vi "Exercise 2.1 DHTxx.vi"() -> ()   [LabVIEW 2014]
uses:
  <vilib>/Q-Wave Systems/QwaveSys RPi Training Package (Demo)/Addons/QwaveSys RPi Training Library.lvlib
  <vilib>/RAFA Solutions/Wooden UI Controls Kit Library Light/Graph/XY Graph.ctl
  <vilib>/RAFA Solutions/Wooden UI Controls Kit Library Light/Wooden UI Controls Kit Library Light.lvlib
  <vilib>/RAFA Solutions/Wooden UI Controls Kit Library Light/Numeric/Numeric Indicator.ctl
  <vilib>/RAFA Solutions/Rainbow Flat UI Controls Kit (Light)/Numeric/Thermometer.ctl
  <vilib>/RAFA Solutions/Rainbow Flat UI Controls Kit (Light)/Rainbow Light.lvlib
  <vilib>/RAFA Solutions/Rainbow Flat UI Controls Kit (Light)/Graph/XY Graph.ctl
panel:
  out "Waveform Chart":sgl(graph) caption="F  Chart 2"
  out "F Meter 2":dbl(knob) scale=0.0..100.0
  out "H & C Graph":T1
  out "C Chart":sgl(graph)
  out "H Meter":T2 scale=0.0..100.0
  out "C Meter":dbl(knob) scale=0.0..40.0
  out "F Meter":T3
  out "C&F Graph":T4
  out "Initial Status":i32
  in  "error in (no error)":errorcluster
  out "error out":errorcluster
  out "Active":bool
  out "f":dbl
  out "c":dbl
  out "h":dbl
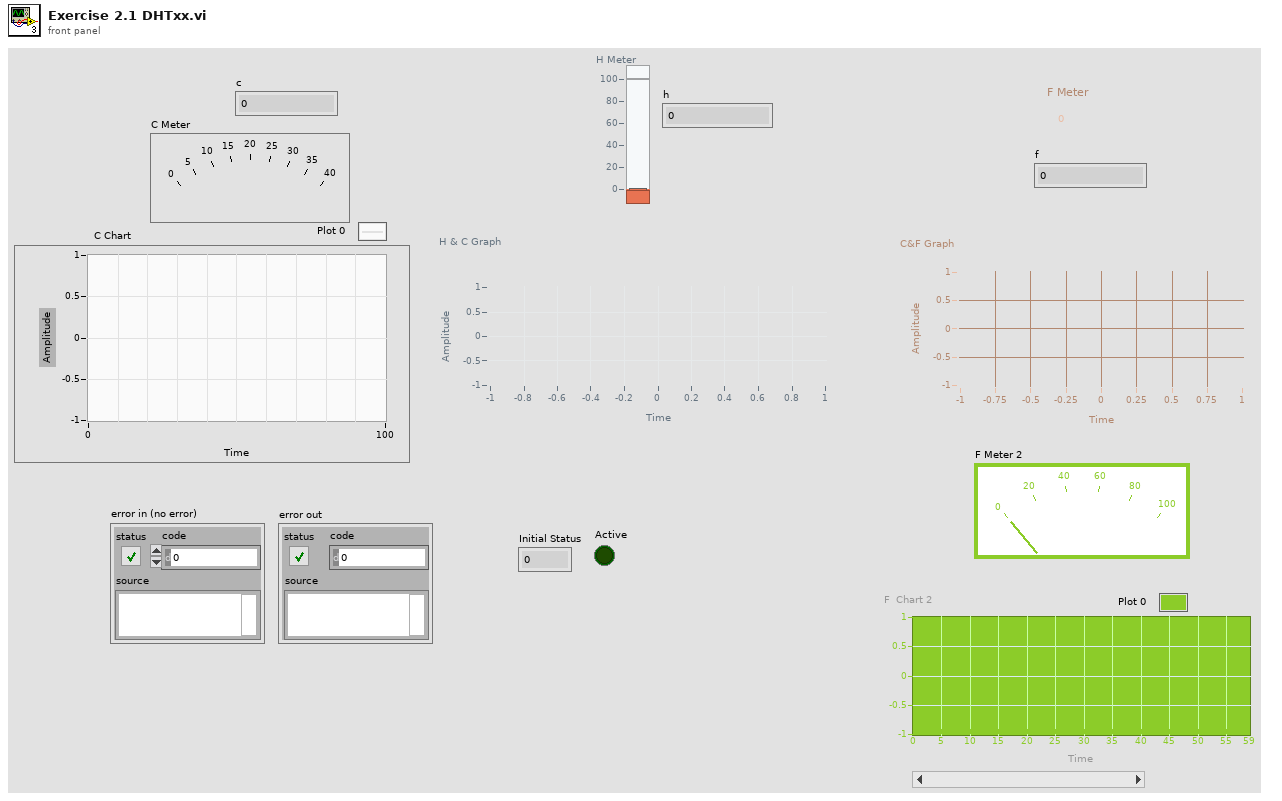
[diagram p1: front panel]
types:
  T1 = typedef "Rainbow Light.lvlib/XY Graph.ctl" = cluster{"X":dbl, "Y":dbl}[]
  T2 = typedef "Rainbow Light.lvlib/Thermometer.ctl" = dbl
  T3 = typedef "Wooden UI Controls Kit Library Light.lvlib/Numeric Indicator.ctl" = dbl
  T4 = typedef "Wooden UI Controls Kit Library Light.lvlib/XY Graph.ctl" = cluster{"X":dbl, "Y":dbl}[]
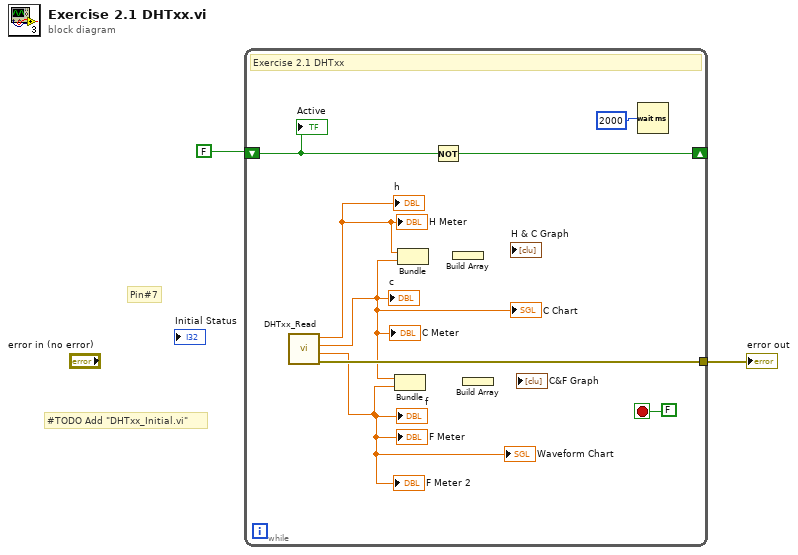
[diagram p0: block diagram]
diagram:
  # "#TODO Add \"DHTxx_Initial.vi\""
  # "Pin#7"
  n1 = while {
    tunnel: [w8] -> w1
    shift-right: [w7] -> _
    shift-left: FALSE -> [w6]
    stop <- FALSE stop-if-true
    # "Exercise 2.1 DHTxx"
    n2 = call <vilib>:"DHTxx_Read.vi"() -> ("error out"=w8:errorcluster, "f"=w3:sgl, "c"=w4:sgl, "h"=w5:sgl)  [unwired: 8 in]
    "h" <- w5
    "c" <- w4
    "f" <- w3
    "C Meter" <- w4
    "C Chart" <- w4
    "H Meter" <- w5
    "F Meter" <- w3
    "F Meter 2" <- w3
    "Waveform Chart" <- w3
    n3 = Bundle("c"=w4, "f"=w3) -> ()  [unwired: 1 in, 1 out]
    n4 = Bundle("h"=w5, "c"=w4) -> ()  [unwired: 1 in, 1 out]
    n5 = Not(x=w6) -> (.not. x?=w7:bool)
    n6 = Build Array "Build Array"() -> ()  [unwired: 1 in, 1 out]
    n7 = Build Array "Build Array"() -> ()  [unwired: 1 in, 1 out]
    n8 = Wait (ms)(milliseconds to wait=u32 2000) -> ()  [unwired: 1 out]
    "Active" <- w6
  }
  "error out" <- w1
